vi "CompilePython.vi"(8 "Stepnum":i32, 9 "Enum":enum16{"Meta", "Aux", "Main"}(ring), 11 "Compiler Settings":T1={"Python Path"=path "", "Main File"="", "Meta File"="", "Aux File"="makesequence.py", "Pre File"="metascript.txt"}) -> (2 "standard output":string, 3 "standard error":string)   [LabVIEW 2019]
uses:
  PulseCompiler/CompilerSettings.ctl
panel:
  out "error out":errorcluster
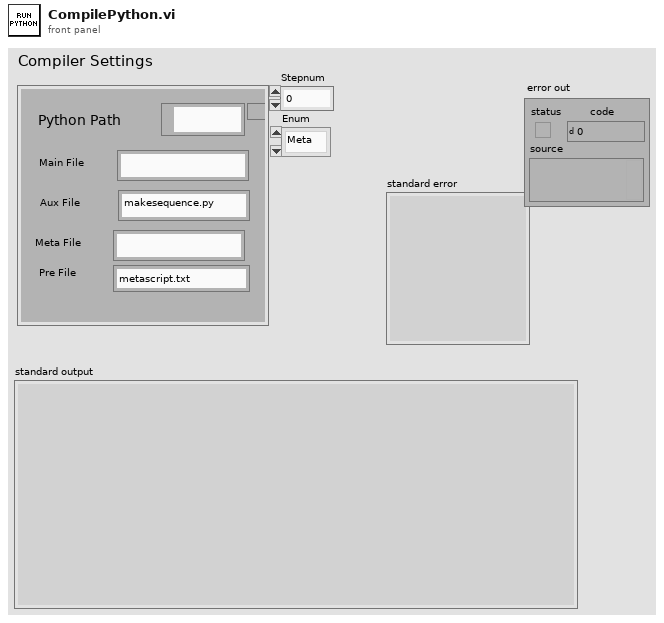
[diagram p1: front panel]
types:
  T1 = typedef "CompilerSettings.ctl" = cluster{"Python Path":path, "Main File":string, "Meta File":string, "Aux File":string, "Pre File":string}
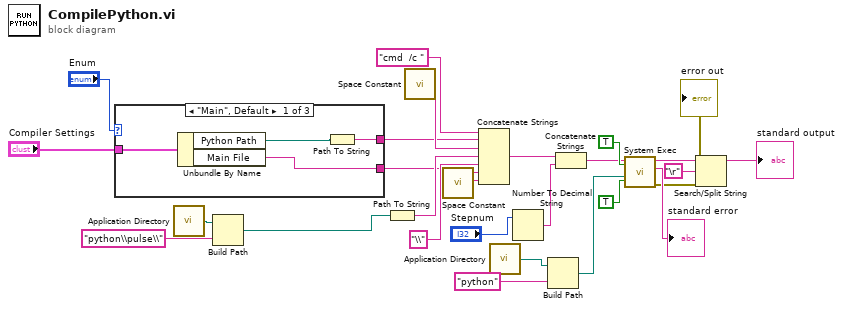
[diagram p0: block diagram]
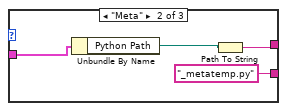
[diagram p2: hidden frame]
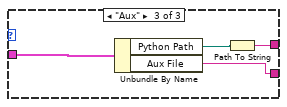
[diagram p3: hidden frame]
diagram:
  n1 = case shown="\"Main\", Default" "Enum" {
    tunnel: [w29 "_metatemp.py" ("Aux File") w37] -> w3
    tunnel: "Compiler Settings" -> [w30 w34 w38]
    tunnel: [w27 w32 w35] -> w1
    frame "Main", Default {
      n2 = Unbundle By Name(w30) -> ("Python Path"=w28:path, "Main File"=w29:string)
      n3 = Path To String(path=w28) -> (string=w27:string)
    }
    frame "Meta" {
      n4 = Unbundle By Name(w34) -> ("Python Path"=w31:path)
      n5 = Path To String(path=w31) -> (string=w32:string)
    }
    frame "Aux" {
      n6 = Unbundle By Name(w38) -> ("Python Path"=w36:path, "Aux File"=w37:string)
      n7 = Path To String(path=w36) -> (string=w35:string)
    }
  }
  n8 = call <vilib>:"Application Directory.vi"() -> ("Application Directory"=w18:path)
  n9 = Build Path(base path=w18, name or relative path="python\\pulse\\") -> (appended path=w20:path)
  n10 = Path To String(path=w20) -> (string=w21:string)
  n11 = call <vilib>:"Space Constant.vi"() -> ("String"=w16:string)
  n12 = call <vilib>:"Space Constant.vi"() -> ("String"=w22:string)
  n13 = Concatenate Strings("cmd  /c " ("string"), w1, w16, w21, "\\" ("string"), w3, w22) -> (w17:string)
  n14 = call <vilib>:"Application Directory.vi"() -> ("Application Directory"=w10:path)
  n15 = Number To Decimal String(number="Stepnum") -> (decimal integer string=w8:string)  [unwired: 1 in]
  n16 = Build Path(base path=w10, name or relative path="python") -> (appended path=w12:path)
  n17 = Concatenate Strings(w17, w8) -> (w9:string)
  n18 = call <vilib>:"System Exec.vi"("run minimized? (F)"=TRUE, "wait until completion? (T)"=TRUE, "working directory"=w12, "command line"=w9) -> ("error out"=→"error out":errorcluster, "standard error"=→"standard error":string, "standard output"=w6:string)  [unwired: 4 in, 1 out]
  n19 = Search/Split String(string=w6, search string/char (-)="\r") -> (substring before match=→"standard output":string)  [unwired: 1 in, 2 out]
